vi "Image Area Calculation.vi"(8 "Error In":errorcluster, 10 "Altitude (m)":dbl, 11 "Camera Settings":T1) -> (0 "Error Out":errorcluster, 1 "Area (m^2)":dbl, 2 "Height (m)":dbl, 3 "Width (m)":dbl)   [LabVIEW 2014]
uses:
  Settings File/Controls/Camera Settings.ctl
panel:
  out "Area (Acres)":dbl
  out "Area (Hectare)":dbl
  out "Area (km^2)":dbl
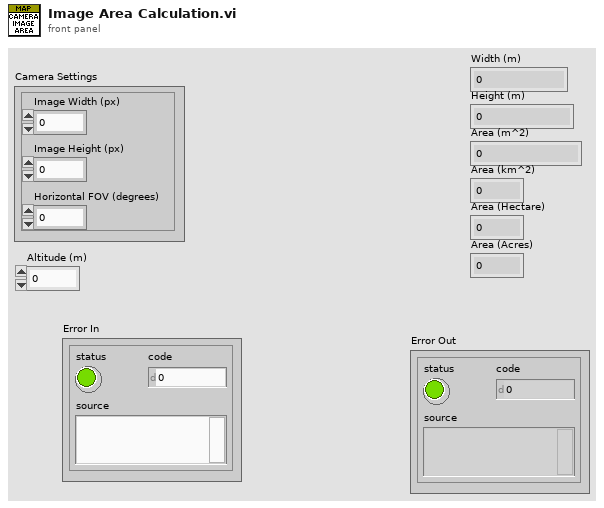
[diagram p1: front panel]
types:
  T1 = typedef "Camera Settings.ctl" = cluster{"Image Width (px)":dbl, "Image Height (px)":dbl, "Horizontal FOV (degrees)":dbl}
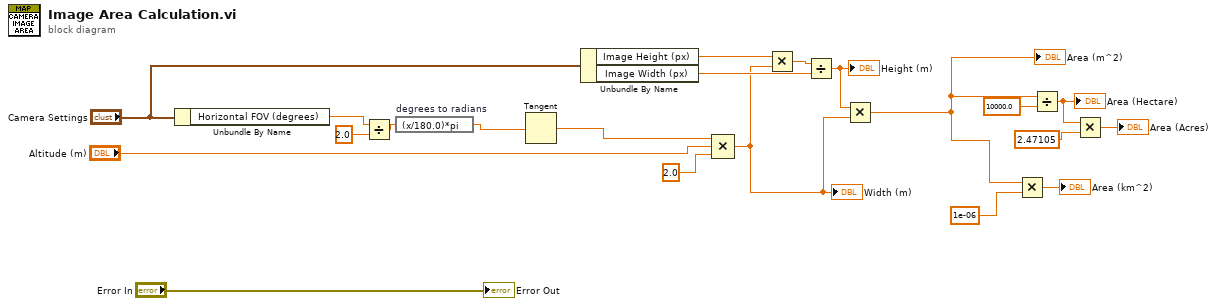
[diagram p0: block diagram]
diagram:
  n1 = Unbundle By Name("Camera Settings") -> ("Horizontal FOV (degrees)"=w12:dbl)
  n2 = Divide(x=w12, y=2.0) -> (x/y=w9:dbl)
  n3 = expression code="(x/180.0)*pi" "degrees to radians"(w9) -> (w11:dbl)
  n4 = Tangent(1:w11) -> (0:w10:dbl)
  n5 = Unbundle By Name("Camera Settings") -> ("Image Height (px)"=w17:dbl, "Image Width (px)"=w16:dbl)
  n6 = Compound Arithmetic op=MULTIPLY(w10, "Altitude (m)", 2.0 ("value")) -> (w13:dbl)
  "Width (m)" <- w13
  n7 = Multiply(x=w17, y=w13) -> (x*y=w15:dbl)
  n8 = Divide(x=w15, y=w16) -> (x/y=w14:dbl)
  "Height (m)" <- w14
  n9 = Multiply(x=w14, y=w13) -> (x*y=w6:dbl)
  "Area (m^2)" <- w6
  n10 = Multiply(x=w6, y=1e-06) -> (x*y=→"Area (km^2)":dbl)
  n11 = Divide(x=w6, y=10000.0) -> (x/y=w4:dbl)
  "Area (Hectare)" <- w4
  n12 = Multiply(x=w4, y=2.47105) -> (x*y=→"Area (Acres)":dbl)
  "Error Out" <- "Error In"
